vi "SendAIProtocol.vi"(7 "Send":bool, 9 "Initialize":bool, 10 "AI prev":T1={"type"="AI", "device"="", "name"="", "data"={"<init"=FALSE, "<avg_bits"=0, "<oversample_bits"=0, ">voltage"=0.0, " Accum Object"={"<init"=FALSE, ">value"=0.0, ">count"=0, "<center"=0, "<deadband"=0}}}, 11 "AI new":T1={"type"="AI", "device"="", "name"="", "data"={"<init"=FALSE, "<avg_bits"=0, "<oversample_bits"=0, ">voltage"=0.0, " Accum Object"={"<init"=FALSE, ">value"=0.0, ">count"=0, "<center"=0, "<deadband"=0}}}) -> ()   [LabVIEW 2019]
uses:
  AI Accum proto.ctl
  AI Data proto.ctl
  AI proto.ctl
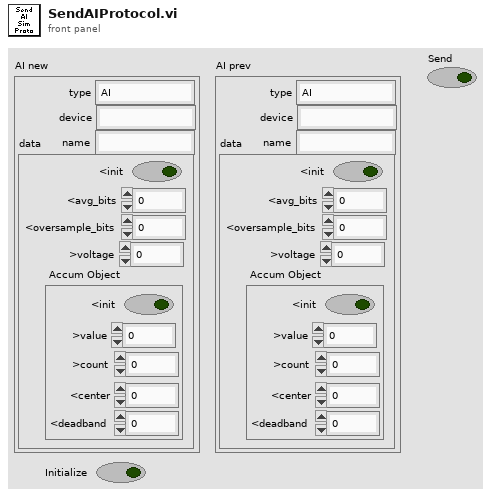
[diagram p1: front panel]
types:
  T1 = typedef "AI proto.ctl" = cluster{"type":string, "device":string, "name":string, "data":T2}
  T2 = typedef "AI Data proto.ctl" = cluster{"<init":bool, "<avg_bits":i32, "<oversample_bits":i32, ">voltage":dbl, " Accum Object":T3}
  T3 = typedef "AI Accum proto.ctl" = cluster{"<init":bool, ">value":dbl, ">count":i32, "<center":i32, "<deadband":i32}
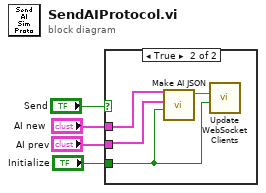
[diagram p0: block diagram]
diagram:
  n1 = case shown="True" "Send" {
    tunnel: "AI new" -> [_ w7]
    tunnel: "AI prev" -> [_ w6]
    tunnel: "Initialize" -> [_ w5]
    frame False {
    }
    frame True {
      n2 = call "Make AI JSON.vi"("Force"=w5, "AI prev"=w6, "AI new"=w7) -> ("delta JSON"=w8:string)  [unwired: 8 in]
      n3 = call "Update WebSocket Clients.vi"("Initialize"=w5, "delta JSON"=w8) -> ()  [unwired: 10 in]
    }
  }
